vi "Query Standard Event Status.vi"(8 "error in (no error)":errorcluster, 11 "VISA resource name":refnum<visa-resource-name>) -> (0 "error out":errorcluster, 2 "Standard Event Status Data Message":string, 3 "VISA resource name out":refnum<visa-resource-name>)   [LabVIEW 2012, in "Stanford Research 830.lvlib"]
doc: "Queries the Standard Event Status register for the Error Data Register group. Essentially, it is used to observe possible invalid results."
uses:
  <instrlib>/Stanford Research 830/Stanford Research 830.lvlib
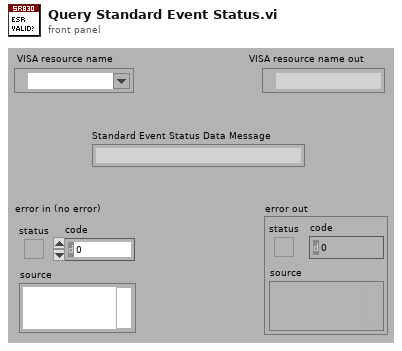
[diagram p1: front panel]
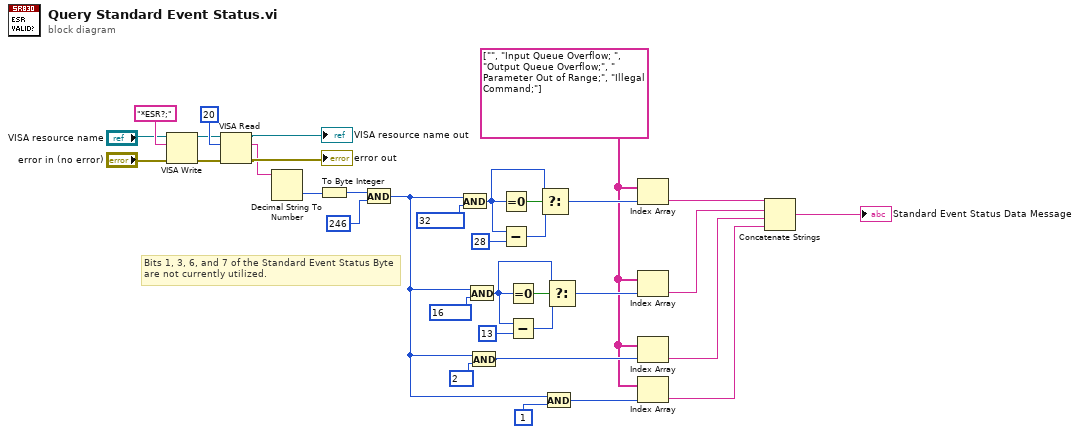
[diagram p0: block diagram]
diagram:
  w11 = string[] ["", "Input Queue Overflow; ", "Output Queue Overflow;", " Parameter Out of Range;", "Illegal Command;"]
  # "Bits 1, 3, 6, and 7 of the Standard Event Status Byte are not currently utilized."
  n1 = VISA Write(VISA resource name="VISA resource name", write buffer="*ESR?;", error in (no error)="error in (no error)") -> (VISA resource name out=w33:refnum<visa-resource-name>, error out=w32:errorcluster)  [unwired: 1 out]
  n2 = VISA Read(VISA resource name=w33, byte count=u32 20, error in (no error)=w32) -> (VISA resource name out=→"VISA resource name out":refnum<visa-resource-name>, read buffer=w2:string, error out=→"error out":errorcluster)  [unwired: 1 out]
  n3 = Decimal String To Number(string=w2) -> (number=w8:i32)  [unwired: 2 in, 1 out]
  n4 = To Byte Integer(number=w8) -> (8bit integer=w1:i8)
  n5 = And(x=w1, y=246) -> (x .and. y?=w5:i32)
  n6 = And(x=w5, y=i8 32) -> (x .and. y?=w22:i32)
  n7 = And(x=w5, y=i8 16) -> (x .and. y?=w17:i32)
  n8 = And(x=w5, y=i8 2) -> (x .and. y?=w12:i32)
  n9 = Equal To 0?(x=w22) -> (x = 0?=w26:bool)
  n10 = Subtract(x=w22, y=28) -> (x-y=w25:i32)
  n11 = Equal To 0?(x=w17) -> (x = 0?=w19:bool)
  n12 = Subtract(x=w17, y=13) -> (x-y=w18:i32)
  n13 = Select(t=w22, s=w26, f=w25) -> (s? t:f=w24:i32)
  n14 = And(x=w5, y=i8 1) -> (x .and. y?=w23:i32)
  n15 = Select(t=w17, s=w19, f=w18) -> (s? t:f=w15:i32)
  n16 = Index Array(array=w11, index=w24) -> (element=w27:string)
  n17 = Index Array(array=w11, index=w15) -> (element=w14:string)
  n18 = Index Array(array=w11, index=w12) -> (element=w10:string)
  n19 = Index Array(array=w11, index=w23) -> (element=w9:string)
  n20 = Concatenate Strings(w27, w14, w10, w9) -> (→"Standard Event Status Data Message":string)
